vi "Read Command _Initialise LCR_.vi"(8 "error in (no error)":errorcluster, 11 "LCRControl in":refnum<class "LCRControl.lvclass">) -> (0 "error out":errorcluster, 2 "Command \"Initialise LCR\"":string, 3 "LCRControl out":refnum<class "LCRControl.lvclass">)   [LabVIEW 2019, in "LCRControl.lvclass"]
uses:
  LCRControl.lvclass
  LCRControl.lvclass/LCRControl.ctl
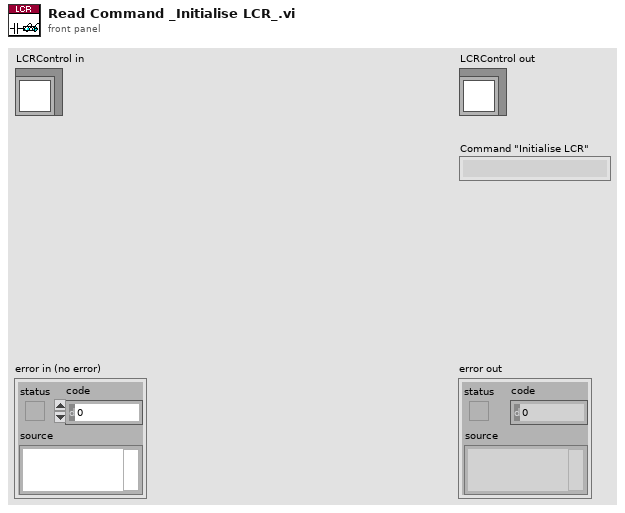
[diagram p1: front panel]
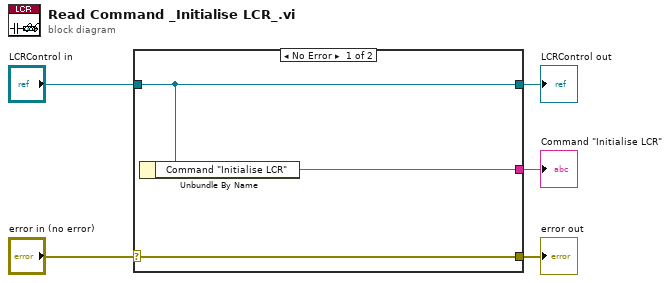
[diagram p0: block diagram]
diagram:
  n1 = case shown="No Error" "error in (no error)" {
    selector: "error in (no error)" -> [w8 w9]
    tunnel: [w8 w9] -> w4
    tunnel: [w7 w10] -> w2
    tunnel: "LCRControl in" -> [w7 w10]
    tunnel: [w6 _] -> w1
    frame No Error {
      n2 = Unbundle By Name(w7) -> ("Command \"Initialise LCR\""=w6:string)
    }
    frame Error {
    }
  }
  "error out" <- w4
  "LCRControl out" <- w2
  "Command \"Initialise LCR\"" <- w1
